vi "ipcamera.vi"() -> ()   [LabVIEW 2018]
uses:
  <vilib>/userdefined/High Color/IMAQdx.ctl
  <vilib>/vision/driver/NI_Vision_Acquisition_Software.lvlib
panel:
  out "IP Camera":T1(plugin-control)
  in  "停止":bool
  in  "Session In":T2
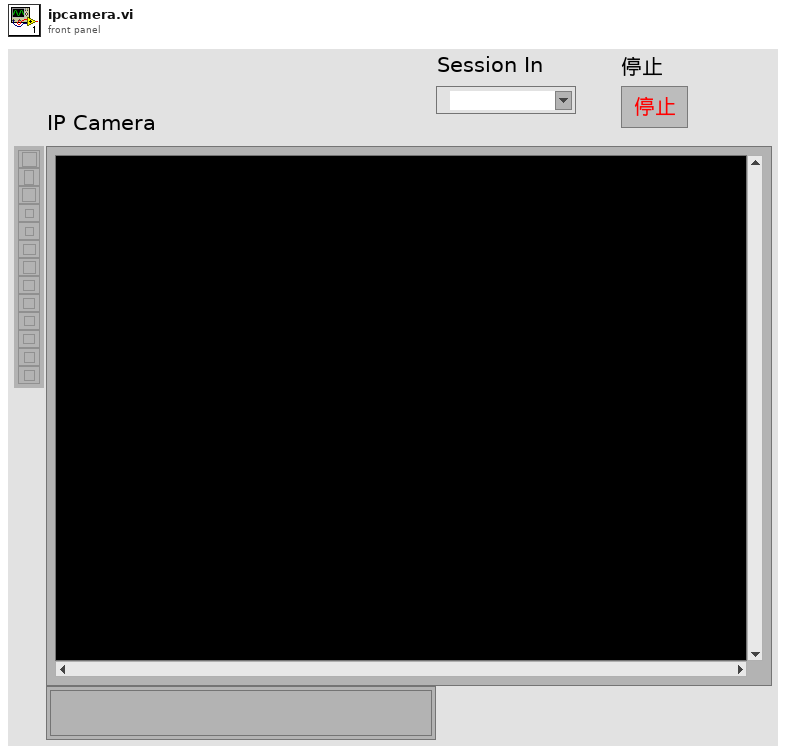
[diagram p1: front panel]
types:
  T1 = typedef "IMAQ Image.ctl" = refnum<image>
  T2 = typedef "IMAQdx.ctl" = refnum<k21>
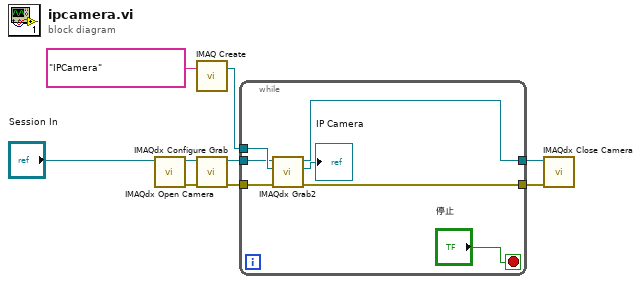
[diagram p0: block diagram]
diagram:
  n1 = call <vilib>:"IMAQdx Open Camera.vi"("Session In"="Session In") -> ("error out"=w6:errorcluster, "Session Out"=w7:T2)  [unwired: 9 in]
  n2 = call "IMAQ Create"("Image Name"="IPCamera") -> ("New Image"=w3:T1)  [unwired: 4 in, 1 out]
  n3 = call <vilib>:"IMAQdx Configure Grab.vi"("error in"=w6, "Session In"=w7) -> ("error out"=w4:errorcluster, "Session Out"=w2:T2)  [unwired: 8 in]
  n4 = while {
    tunnel: [w15] -> w5
    tunnel: w4 -> [w14]
    tunnel: w3 -> [w13]
    tunnel: w2 -> [w12]
    tunnel: [w10] -> w1
    stop <- "停止" stop-if-true
    n5 = call <vilib>:"IMAQdx Grab2.vi"("error in"=w14, "Image In"=w13, "Session In"=w12) -> ("error out"=w15:errorcluster, "Image Out"=→"IP Camera":T1, "Session Out"=w10:T2)  [unwired: 5 in, 1 out]
  }
  n6 = call <vilib>:"IMAQdx Close Camera.vi"("error in"=w5, "Session In"=w1) -> ()  [unwired: 9 in, 1 out]
